vi "Refresh Palettes.vi"   [LabVIEW 2017]
doc: "Updates the Controls and Functions palette set programmatically.\n\nThis method is similar to the <B>Save Changes</B> button on the Edit Controls and Functions Palette Set dialog box."
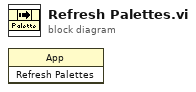
[diagram p0: block diagram]
diagram:
  n1 = invoke class="App" method="Refresh Palettes"() -> ()  [unwired: 3 in, 3 out]
